vi "Get Configuration.vi"(11 "error in (no error)":errorcluster) -> (4 "Config":string, 15 "error out":errorcluster)   [LabVIEW 2024, in "GRBL 1.1.lvlib"]
doc: "Get the complete list of current configuration ni the selected controler"
uses:
  GRBL 1.1.lvlib
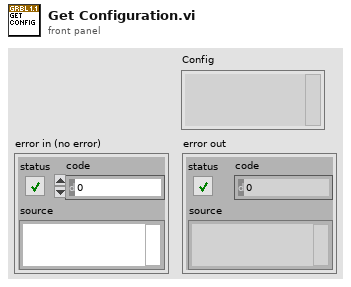
[diagram p1: front panel]
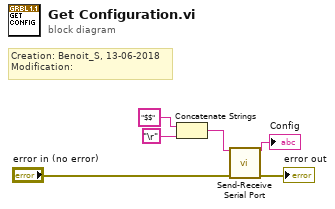
[diagram p0: block diagram]
diagram:
  # "Creation: Benoit_S, 13-06-2018\nModification:"
  n1 = Concatenate Strings("$$", "\r") -> (w5:string)
  n2 = call "Send-Receive Serial Port.vi"("Data to write"=w5, "error in (no error)"="error in (no error)") -> ("Data read"=→"Config":string, "error out"=→"error out":errorcluster)  [unwired: 12 in]
